vi "Progress Bar.vi"(5 "Total Number":dbl, 9 "Current Number":dbl) -> (8 "Scan Progress":dbl(slide) caption="Slide" scale=0.0..100.0)   [LabVIEW 2013]
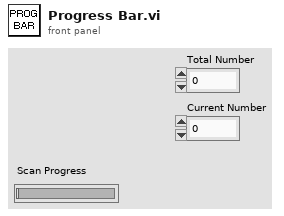
[diagram p1: front panel]
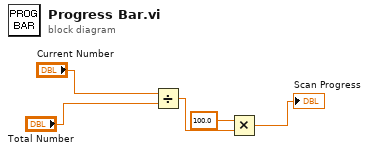
[diagram p0: block diagram]
diagram:
  n1 = Divide(x="Current Number", y="Total Number") -> (x/y=w3:dbl)
  n2 = Multiply(x=100.0, y=w3) -> (x*y=→"Scan Progress":dbl)
